vi "ACDC_Config_9234.vi"(8 "error in (no error)":errorcluster, 9 "Input Config Array":T1[](array[typedef])=[0, 0, 0, 0, 0, 0, 0, 0, 0, 0, 0, 0, 0, 0, 0, 0, 0, 0, 0, 0, 0, 0, 0, 0, 0, 0, 0, 0, 0, 0, 0, 0] items=["AC Coupled", "DC Coupled", "IEPE AC Coupled"], 10 "Data Rate [S/s]":u32) -> (0 "error out":errorcluster)   [LabVIEW 2017, in "BOP_VibAPI_6.lvlib"]
uses:
  <vilib>/addons/InsightCM/Devices/Shared/Cms/Fpga/Acquisition/source/subVIs/VibAPI/BOP_VibAPI_6.lvlib
  <vilib>/LabVIEW Targets/FPGA/cRIO/shared/nicrio_ModuleControls/nicrio_cRIO-9232_ConfigModeRing.ctl
  <vilib>/rvi/eio/common/nirviEmuTemplatePropertySet_errors.vi
  <vilib>/eio/EIOPropertyNode/EIOPropertyNode.xnode
  <vilib>/LabVIEW Targets/FPGA/cRIO/shared/nicrio_ModuleControls/nicrio_cRIO-9234_DataRatesRing2.ctl
  <vilib>/LabVIEW Targets/FPGA/cRIO/shared/nicrio_ModuleControls/nicrio_cRIO-9234_ConfigModeRing.ctl
  <vilib>/rvi/eio/common/nirviEmuTemplatePropertyGet_errors.vi
  <vilib>/rvi/eio/common/nirviEmuTemplatePropertyGet_noerrors.vi
  <vilib>/rvi/eio/common/nirviEmuTemplatePropertySet_noerrors.vi
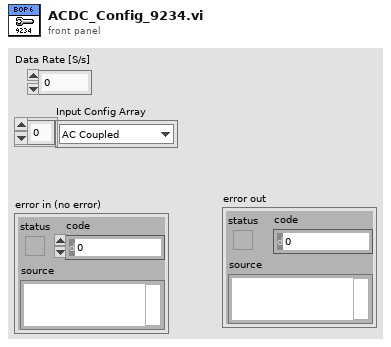
[diagram p1: front panel]
types:
  T1 = typedef "nicrio_cRIO-9232_ConfigModeRing.ctl" = u8
  T2 = typedef "nicrio_cRIO-9234_DataRatesRing2.ctl" = u8
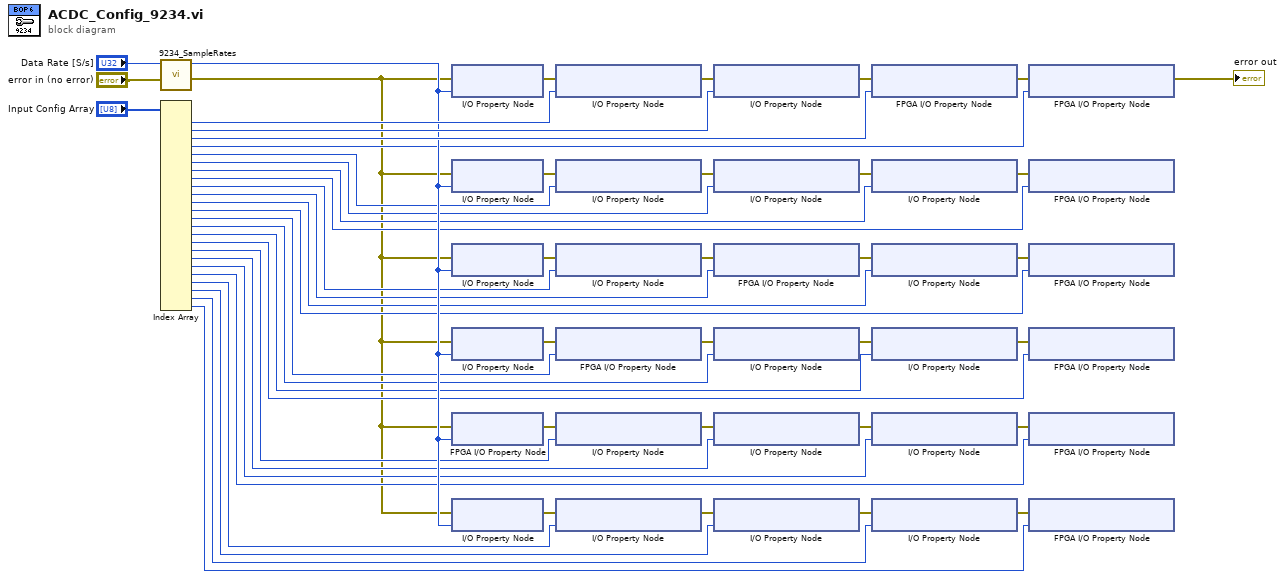
[diagram p0: block diagram]
diagram:
  n1 = call <vilib>:"9234_SampleRates.vi"("error in (no error)"="error in (no error)", "Data Rate [S/s]"="Data Rate [S/s]") -> ("error out"=w1:errorcluster, "Data Rate"=w31:T2)  [unwired: 8 in]
  n2 = Index Array(array="Input Config Array") -> (element #1=w46:T1, element #2=w45:T1, element #3=w44:T1, element #4=w2:T1, element #5=w3:T1, element #6=w4:T1, element #7=w5:T1, element #8=w6:T1, element #9=w7:T1, element #10=w8:T1, element #11=w9:T1, element #12=w10:T1, element #13=w11:T1, element #14=w12:T1, element #15=w13:T1, element #16=w14:T1, element #17=w15:T1, element #18=w16:T1, element #19=w17:T1, element #20=w18:T1, element #21=w19:T1, element #22=w20:T1, element #23=w21:T1, element #24=w22:T1)  [unwired: 24 in]
  n3 = xnode "I/O Property Node"("error in"=w1, "Data Rate"=w31) -> ("error out"=w48:errorcluster)  [unwired: 1 in, 1 out]
  n4 = xnode "I/O Property Node"("error in"=w1, "Data Rate"=w31) -> ("error out"=w47:errorcluster)  [unwired: 1 in, 1 out]
  n5 = xnode "I/O Property Node"("error in"=w1, "Data Rate"=w31) -> ("error out"=w43:errorcluster)  [unwired: 1 in, 1 out]
  n6 = xnode "I/O Property Node"("error in"=w1, "Data Rate"=w31) -> ("error out"=w38:errorcluster)  [unwired: 1 in, 1 out]
  n7 = xnode "FPGA I/O Property Node"("error in"=w1, "Data Rate"=w31) -> ("error out"=w37:errorcluster)  [unwired: 1 in, 1 out]
  n8 = xnode "I/O Property Node"("error in"=w1, "Data Rate"=w31) -> ("error out"=w32:errorcluster)  [unwired: 1 in, 1 out]
  n9 = xnode "I/O Property Node"("error in"=w48, "Input Configuration"=w46) -> ("error out"=w49:errorcluster)  [unwired: 1 in, 1 out]
  n10 = xnode "I/O Property Node"("error in"=w47, "Input Configuration"=w3) -> ("error out"=w51:errorcluster)  [unwired: 1 in, 1 out]
  n11 = xnode "I/O Property Node"("error in"=w43, "Input Configuration"=w7) -> ("error out"=w42:errorcluster)  [unwired: 1 in, 1 out]
  n12 = xnode "FPGA I/O Property Node"("error in"=w38, "Input Configuration"=w11) -> ("error out"=w39:errorcluster)  [unwired: 1 in, 1 out]
  n13 = xnode "I/O Property Node"("error in"=w37, "Input Configuration"=w15) -> ("error out"=w36:errorcluster)  [unwired: 1 in, 1 out]
  n14 = xnode "I/O Property Node"("error in"=w32, "Input Configuration"=w19) -> ("error out"=w33:errorcluster)  [unwired: 1 in, 1 out]
  n15 = xnode "I/O Property Node"("error in"=w49, "Input Configuration"=w45) -> ("error out"=w50:errorcluster)  [unwired: 1 in, 1 out]
  n16 = xnode "I/O Property Node"("error in"=w51, "Input Configuration"=w4) -> ("error out"=w52:errorcluster)  [unwired: 1 in, 1 out]
  n17 = xnode "FPGA I/O Property Node"("error in"=w42, "Input Configuration"=w8) -> ("error out"=w41:errorcluster)  [unwired: 1 in, 1 out]
  n18 = xnode "I/O Property Node"("error in"=w39, "Input Configuration"=w12) -> ("error out"=w40:errorcluster)  [unwired: 1 in, 1 out]
  n19 = xnode "I/O Property Node"("error in"=w36, "Input Configuration"=w16) -> ("error out"=w35:errorcluster)  [unwired: 1 in, 1 out]
  n20 = xnode "I/O Property Node"("error in"=w33, "Input Configuration"=w20) -> ("error out"=w34:errorcluster)  [unwired: 1 in, 1 out]
  n21 = xnode "FPGA I/O Property Node"("error in"=w50, "Input Configuration"=w44) -> ("error out"=w29:errorcluster)  [unwired: 1 in, 1 out]
  n22 = xnode "I/O Property Node"("error in"=w52, "Input Configuration"=w5) -> ("error out"=w28:errorcluster)  [unwired: 1 in, 1 out]
  n23 = xnode "I/O Property Node"("error in"=w41, "Input Configuration"=w9) -> ("error out"=w27:errorcluster)  [unwired: 1 in, 1 out]
  n24 = xnode "I/O Property Node"("error in"=w40, "Input Configuration"=w13) -> ("error out"=w25:errorcluster)  [unwired: 1 in, 1 out]
  n25 = xnode "I/O Property Node"("error in"=w35, "Input Configuration"=w17) -> ("error out"=w24:errorcluster)  [unwired: 1 in, 1 out]
  n26 = xnode "I/O Property Node"("error in"=w34, "Input Configuration"=w21) -> ("error out"=w23:errorcluster)  [unwired: 1 in, 1 out]
  n27 = xnode "FPGA I/O Property Node"("error in"=w29, "Input Configuration"=w2) -> ("error out"=→"error out":errorcluster)  [unwired: 1 in, 1 out]
  n28 = xnode "FPGA I/O Property Node"("error in"=w28, "Input Configuration"=w6) -> ()  [unwired: 1 in, 2 out]
  n29 = xnode "FPGA I/O Property Node"("error in"=w27, "Input Configuration"=w10) -> ()  [unwired: 1 in, 2 out]
  n30 = xnode "FPGA I/O Property Node"("error in"=w25, "Input Configuration"=w14) -> ()  [unwired: 1 in, 2 out]
  n31 = xnode "FPGA I/O Property Node"("error in"=w24, "Input Configuration"=w18) -> ()  [unwired: 1 in, 2 out]
  n32 = xnode "FPGA I/O Property Node"("error in"=w23, "Input Configuration"=w22) -> ()  [unwired: 1 in, 2 out]
